vi "Serial Comms - Establish Connection.vi"(8 "error in (no error)":errorcluster, 11 "Serial Comms in":refnum<class "Serial Comms.lvclass">) -> (0 "error out":errorcluster, 3 "Serial Comms out":refnum<class "Serial Comms.lvclass">)   [LabVIEW 2020, in "Generic_Comms.lvlib" / "Serial Comms.lvclass"]
uses:
  Serial Comms.lvclass
  Serial Comms.lvclass/Serial Comms.ctl
  <vilib>/Instr/_visa.llb/VISA Configure Serial Port (Instr).vi
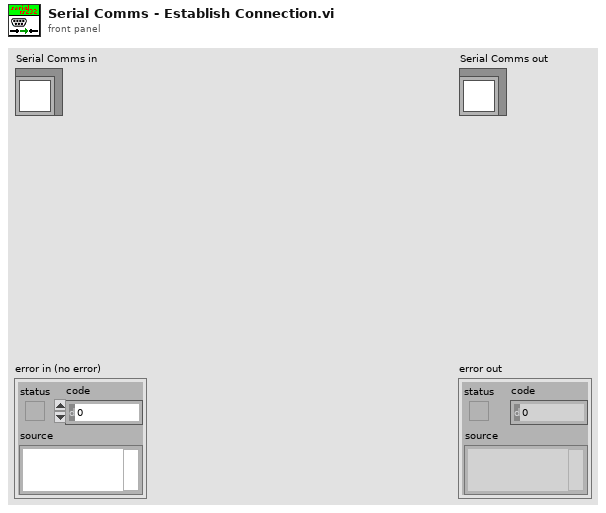
[diagram p1: front panel]
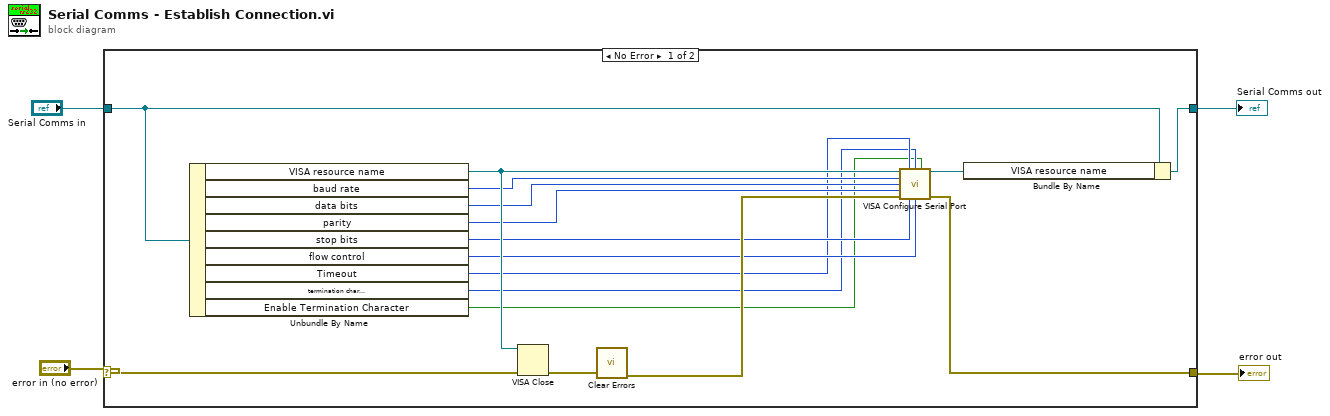
[diagram p0: block diagram]
diagram:
  n1 = case shown="No Error" "error in (no error)" {
    selector: "error in (no error)" -> [w20 w22]
    tunnel: [w8 w22] -> w3
    tunnel: [w6 w21] -> w1
    tunnel: "Serial Comms in" -> [w7 w21]
    frame No Error {
      n2 = Unbundle By Name(w7) -> ("VISA resource name"=w18:refnum<visa-resource-name>, "baud rate"=w16:u32, "data bits"=w15:u16, "parity"=w14:enum16{"None", "Odd", "Even", "Mark", "Space"}, "stop bits"=w13:u16, "flow control"=w12:u16, "Timeout"=w11:u32, "termination char\n(0xA = '\\n' = LF)"=w10:u8, "Enable Termination Character"=w9:bool)
      n3 = VISA Close(VISA resource name=w18, error in (no error)=w20) -> (error out=w19:errorcluster)
      n4 = call <vilib>:"Clear Errors.vi"("error in (no error)"=w19) -> ("error out"=w17:errorcluster)  [unwired: 5 in, 1 out]
      n5 = call-poly "VISA Configure Serial Port"("VISA resource name"=w18, "timeout (10sec)"=w11, "termination char\n(0xA = '\\n' = LF)"=w10, "Enable Termination\nChar (T)"=w9, "baud rate (9600)"=w16, "data bits (8)"=w15, "parity (0:none)"=w14, "error in (no error)"=w17, "stop bits (10: 1 bit)"=w13, "flow control (0:none)"=w12) -> ("VISA resource name out"=w5:refnum<visa-resource-name>, "error out"=w8:errorcluster)  [unwired: 4 out]
      n6 = Bundle By Name(cluster=w7, "VISA resource name"=w5) -> (w6:refnum<class "Serial Comms.lvclass">)
    }
    frame Error {
    }
  }
  "error out" <- w3
  "Serial Comms out" <- w1
